vi "Get point.vi"(8 "error in (no error)":errorcluster, 11 "IV in":refnum<class "IV.lvclass">) -> (0 "error out":errorcluster, 1 "y":dbl, 2 "x":dbl, 3 "IV out":refnum<class "IV.lvclass">)   [LabVIEW 2014, in "IV.lvclass"]
uses:
  IV.lvclass
  data/IV_data.lvclass
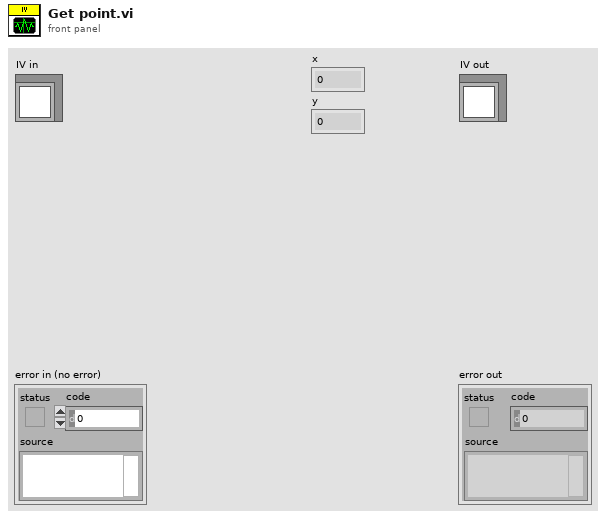
[diagram p1: front panel]
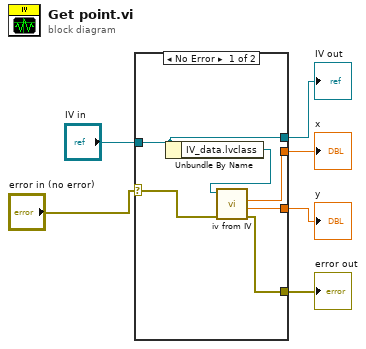
[diagram p0: block diagram]
diagram:
  n1 = case shown="No Error" "error in (no error)" {
    selector: "error in (no error)" -> [w9 w14]
    tunnel: "IV in" -> [w7 w13]
    tunnel: [w11 _] -> w4
    tunnel: [w10 _] -> w3
    tunnel: [w8 w14] -> w2
    tunnel: [w7 w13] -> w1
    frame No Error {
      n2 = Unbundle By Name(w7) -> ("IV_data.lvclass"=w12:refnum<class "IV_data.lvclass">)
      n3 = call-dynamic "iv from IV.vi"("error in (no error)"=w9, "IV_data in"=w12) -> ("error out"=w8:errorcluster, "y"=w10:dbl, "x"=w11:dbl)  [unwired: 6 in, 1 out]
    }
    frame Error {
    }
  }
  "error out" <- w2
  "IV out" <- w1
  "y" <- w3
  "x" <- w4
